vi "toado (SubVI).vi"(9 "X3":dbl, 10 "X2":dbl, 11 "X1":dbl) -> (2 "Y_ph":dbl, 3 "X_ph":dbl)   [LabVIEW 2019]
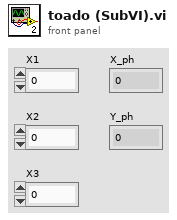
[diagram p1: front panel]
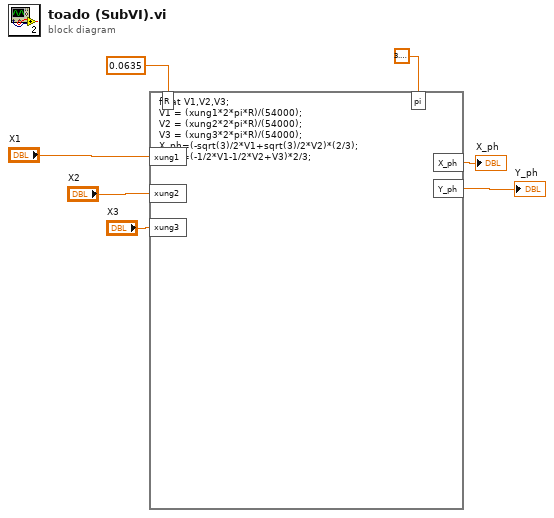
[diagram p0: block diagram]
diagram:
  n1 = formula code="float V1,V2,V3;\nV1 = (xung1*2*pi*R)/(54000);\nV2 = (xung2*2*pi*R)/(54000);\nV3 = (xung3*2*pi*R)/(54000);\nX_ph=(-sqrt(3)/2*V1+sqrt(3)/2*V2)*(2/3);\nY_ph=(-1/2*V1-1/2*V2+V3)*2/3;"("xung1"="X1", "xung2"="X2", "xung3"="X3", "pi"=3.141592653589793, "R"=0.0635 ("input variable")) -> ("X_ph"=→"X_ph":dbl, "Y_ph"=→"Y_ph":dbl)
